vi "v5.5.vi"() -> ()   [LabVIEW 2018]
uses:
  <vilib>/DAQmx/read.llb/DAQmx Read (Analog 1D DBL NChan 1Samp).vi
  <extravilib>/ChannelInstances/Lossy Stream-c(a[.](c(dbl,dbl,dbl,dbl)),stamp,a[.](dbl),c(dbl,dbl,dbl,dbl,dbl,dbl,dbl))/Read With Abort.vi
  <extravilib>/ChannelInstances/High Speed Stream-c(a[.](c(dbl,dbl,dbl,dbl)),stamp,a[.](dbl),c(dbl,dbl,dbl,dbl,dbl,dbl,dbl))/_Read For Replicate.vi
  <extravilib>/ChannelInstances/Lossy Stream-c(a[.](c(dbl,dbl,dbl,dbl)),stamp,a[.](dbl),c(dbl,dbl,dbl,dbl,dbl,dbl,dbl))/Write With Abort.vi
  <extravilib>/ChannelInstances/Lossy Stream-c(a[.](c(dbl,dbl,dbl,dbl)),stamp,a[.](dbl),c(dbl,dbl,dbl,dbl,dbl,dbl,dbl))/EndpointRead.vi
  <extravilib>/ChannelInstances/Lossy Stream-c(a[.](c(dbl,dbl,dbl,dbl)),stamp,a[.](dbl),c(dbl,dbl,dbl,dbl,dbl,dbl,dbl))/Endpoint.vi
  <extravilib>/ChannelInstances/Lossy Stream-c(a[.](c(dbl,dbl,dbl,dbl)),stamp,a[.](dbl),c(dbl,dbl,dbl,dbl,dbl,dbl,dbl))/Instantiate.vi
  <extravilib>/ChannelInstances/Lossy Stream-c(a[.](c(dbl,dbl,dbl,dbl)),stamp,a[.](dbl),c(dbl,dbl,dbl,dbl,dbl,dbl,dbl))/)Channel.vi
  <resource>/ChannelSupport/_ChannelSupport/WaitIfNeeded.vi
  <extravilib>/ChannelInstances/High Speed Stream-c(a[.](c(dbl,dbl,dbl,dbl)),stamp,a[.](dbl),c(dbl,dbl,dbl,dbl,dbl,dbl,dbl))/Instantiate.vi
  <extravilib>/ChannelInstances/High Speed Stream-c(a[.](c(dbl,dbl,dbl,dbl)),stamp,a[.](dbl),c(dbl,dbl,dbl,dbl,dbl,dbl,dbl))/)Channel.vi
  <extravilib>/ChannelInstances/High Speed Stream-c(a[.](c(dbl,dbl,dbl,dbl)),stamp,a[.](dbl),c(dbl,dbl,dbl,dbl,dbl,dbl,dbl))/Abort Signal/Init Signal.vi
  <vilib>/Utility/file.llb/Write Delimited Spreadsheet (string).vi
  <vilib>/DAQmx/create/channels.llb/DAQmx Create Channel (AI-Temperature-Thermocouple).vi
  <vilib>/DAQmx/configure/timing.llb/DAQmx Timing (Sample Clock).vi
  <vilib>/DAQmx/miscellaneous.llb/DAQmx Fill In Error Info.vi
  <extravilib>/ChannelInstances/High Speed Stream-c(a[.](c(dbl,dbl,dbl,dbl)),stamp,a[.](dbl),c(dbl,dbl,dbl,dbl,dbl,dbl,dbl)).lvlib
  <resource>/objmgr/daqmx.rc
  <extravilib>/ChannelInstances/Lossy Stream-c(a[.](c(dbl,dbl,dbl,dbl)),stamp,a[.](dbl),c(dbl,dbl,dbl,dbl,dbl,dbl,dbl)).lvlib
panel:
  out "Equivalence Ratio":dbl
  out "Total Air Flow Required for Stoichiometric Combustion":dbl
  out "Mixture AFR":dbl
  out "Total Fuel Flow [g/s]":dbl
  out "Total Air Flow [g/s]":dbl
  in  "Rig Temperature Tab Box":enum32{"Rig Temps Live", "Alarm Thresholds"}(tab)
  out "Rig Temperatures":T1
  in  "Rig Alarm Thresholds":T1
  out "DAQ Current Time":timestamp format="%<%X>T"
  in  "UI Refresh Rate (Hz)":u32=1 min=1 max=500 step=1
  out "Line Pressures":T2(graph)
  in  "Boondoggle":dbl(slide) scale=0.0..10.0
  out "Line Temperatures":T2(graph)
  in  "Species List":string[][](table)=[["Custom", "9999999999"], ["Methanol", "6.47"], ["Butanol", "11.2"], ["Diesel", "14.5"], ["Gasoline", "14.7"], ["Propane", "15.67"], ["Methane", "13.19"], ["Hydrogen", "34.3"], ["Ammonia", "6.0466"], ["Pentane", "15.32"], ["Butane", "14.98"], ["Hexane", "15.24"], ["Ethanol", "9"], ["Empty (Not Used)", "0"]]
  in  "Lines Tab Control\n(Don't delete)":enum32{"Live Data", "AFR Info", "Setup Lines"}(tab)
  out "Flowrate Data":T3(array[cluster])
  out "AFR Display":T4(array[cluster])
  in  "Line Setup":T5(array[cluster])
  out "Actual Sample Rate":dbl
  out "Export Timestamp":timestamp format="%<%H:%M:%S>T"
  out "UI Timestamp":timestamp format="%<%X\n%x>T"
  in  "file path (dialog if empty)":path
  out "Export Loop Status":T6(ring)
  in  "Start Recording?":bool
  in  "Stop Recording?":bool
  out "Aquisition\nLoop Status":T7(ring)
  in  "OK Button":bool
  in  "DAQ Properties":cluster{"Sample Rate [Hz]":dbl}={"Sample Rate [Hz]"=1.0} {"Sample Rate [Hz]" min=1.0 max=500.0 step=1.0}
  # "Rig Temperatures [ °C]"
  # "Rig Alarm Thresholds [ °C]"
  # "Live \n Live Line Data"
  # "Air-to-Fuel Ratios for each Line"
  # "Line Setup"
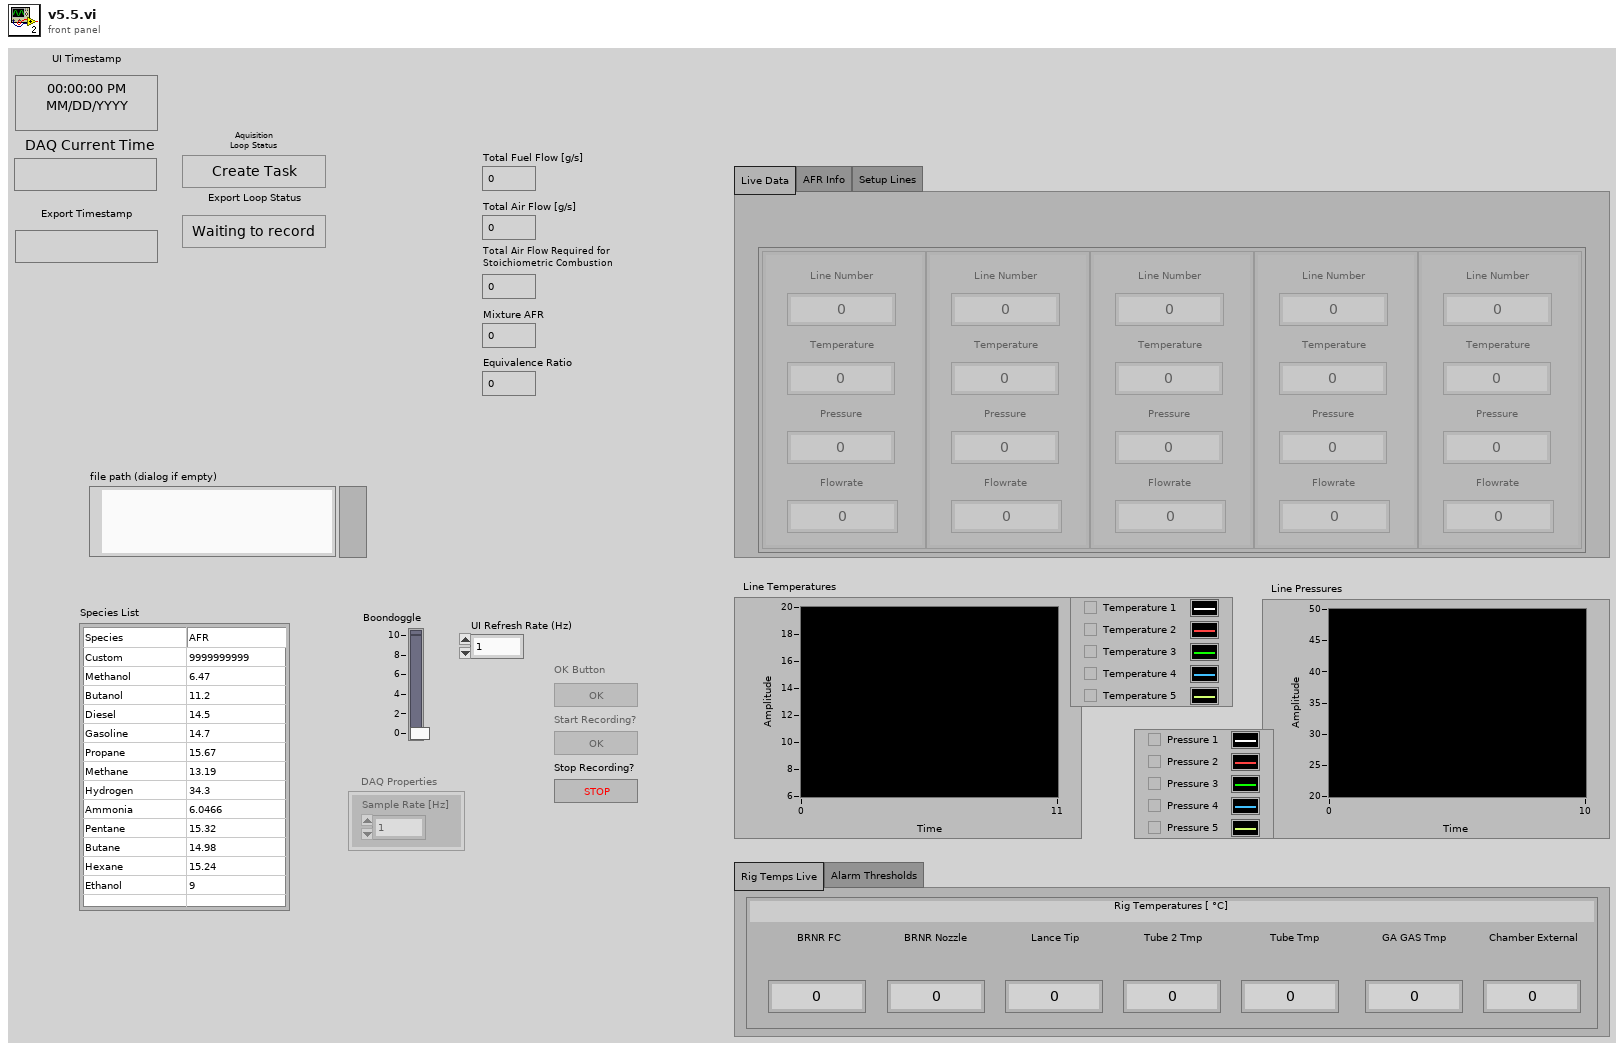
[diagram p1: front panel]
types:
  T1 = cluster{"BRNR FC":dbl, "BRNR Nozzle":dbl, "Lance Tip":dbl, "Tube 2 Tmp":dbl, "Tube Tmp":dbl, "GA GAS Tmp":dbl, "Chamber External":dbl}
  T2 = cluster{"[0]":dbl, "[1]":dbl, "[2]":dbl, "[3]":dbl, "[4]":dbl}
  T3 = cluster{"Line Number":dbl, "Temperature":dbl, "Pressure":dbl, "Flowrate":dbl}[]
  T4 = cluster{"Line Number":i32, "AFR":dbl, "Species":enum16{"Empty (Not used)", "Custom", "Air", "Methanol", "Ethanol", "Butanol", "Diesel", "Gasoline", "Propane", "Methane", "Hydrogen", "Pentane", "Butane", "Hexane"}}[]
  T5 = cluster{"Custom AFR":dbl, "Species":enum16{"Empty (Not used)", "Custom", "Air", "Methanol", "Ethanol", "Butanol", "Diesel", "Gasoline", "Propane", "Methane", "Hydrogen", "Pentane", "Butane", "Hexane"}}[]
  T6 = enum16{"Waiting to record", "Creating Spreadsheet", "Recording", "Finished Recording"}
  T7 = enum16{"Create Task", "Change Settings", "Check Settings", "Read Data", "End Task"}
  T8 = enum8{"Enabled", "Disabled", "Disabled and Grayed Out"}
  T9 = cluster{"Flowrate Data":cluster{"Line Number":dbl, "Temperature":dbl, "Pressure":dbl, "Flowrate":dbl}[], "Current Time":timestamp, "DAQmx Data":dbl[], "Rig Temperatures":cluster{"BRNR FC":dbl, "BRNR Nozzle":dbl, "Lance Tip":dbl, "Tube 2 Tmp":dbl, "Tube Tmp":dbl, "GA GAS Tmp":dbl, "Chamber External Temp":dbl}}
  T10 = cluster{"BRNR FC":dbl, "BRNR Nozzle":dbl, "Lance Tip":dbl, "Tube 2 Tmp":dbl, "Tube Tmp":dbl, "GA GAS Tmp":dbl, "Chamber External Temp":dbl}
  T11 = typedef "High Speed Stream-c(a[.](c(dbl,dbl,dbl,dbl)),stamp,a[.](dbl),c(dbl,dbl,dbl,dbl,dbl,dbl,dbl)).lvlib/)Channel.ctl" = refnum<queue>
  T12 = typedef "Lossy Stream-c(a[.](c(dbl,dbl,dbl,dbl)),stamp,a[.](dbl),c(dbl,dbl,dbl,dbl,dbl,dbl,dbl)).lvlib/)Channel.ctl" = refnum<queue>
  T13 = cluster{"Line":i32, "AFR":dbl, "Species":enum16{"Empty (Not used)", "Custom", "Air", "Methanol", "Ethanol", "Butanol", "Diesel", "Gasoline", "Propane", "Methane", "Hydrogen", "Pentane", "Butane", "Hexane"}}
  T14 = enum16{"Empty (Not used)", "Custom", "Air", "Methanol", "Ethanol", "Butanol", "Diesel", "Gasoline", "Propane", "Methane", "Hydrogen", "Pentane", "Butane", "Hexane"}
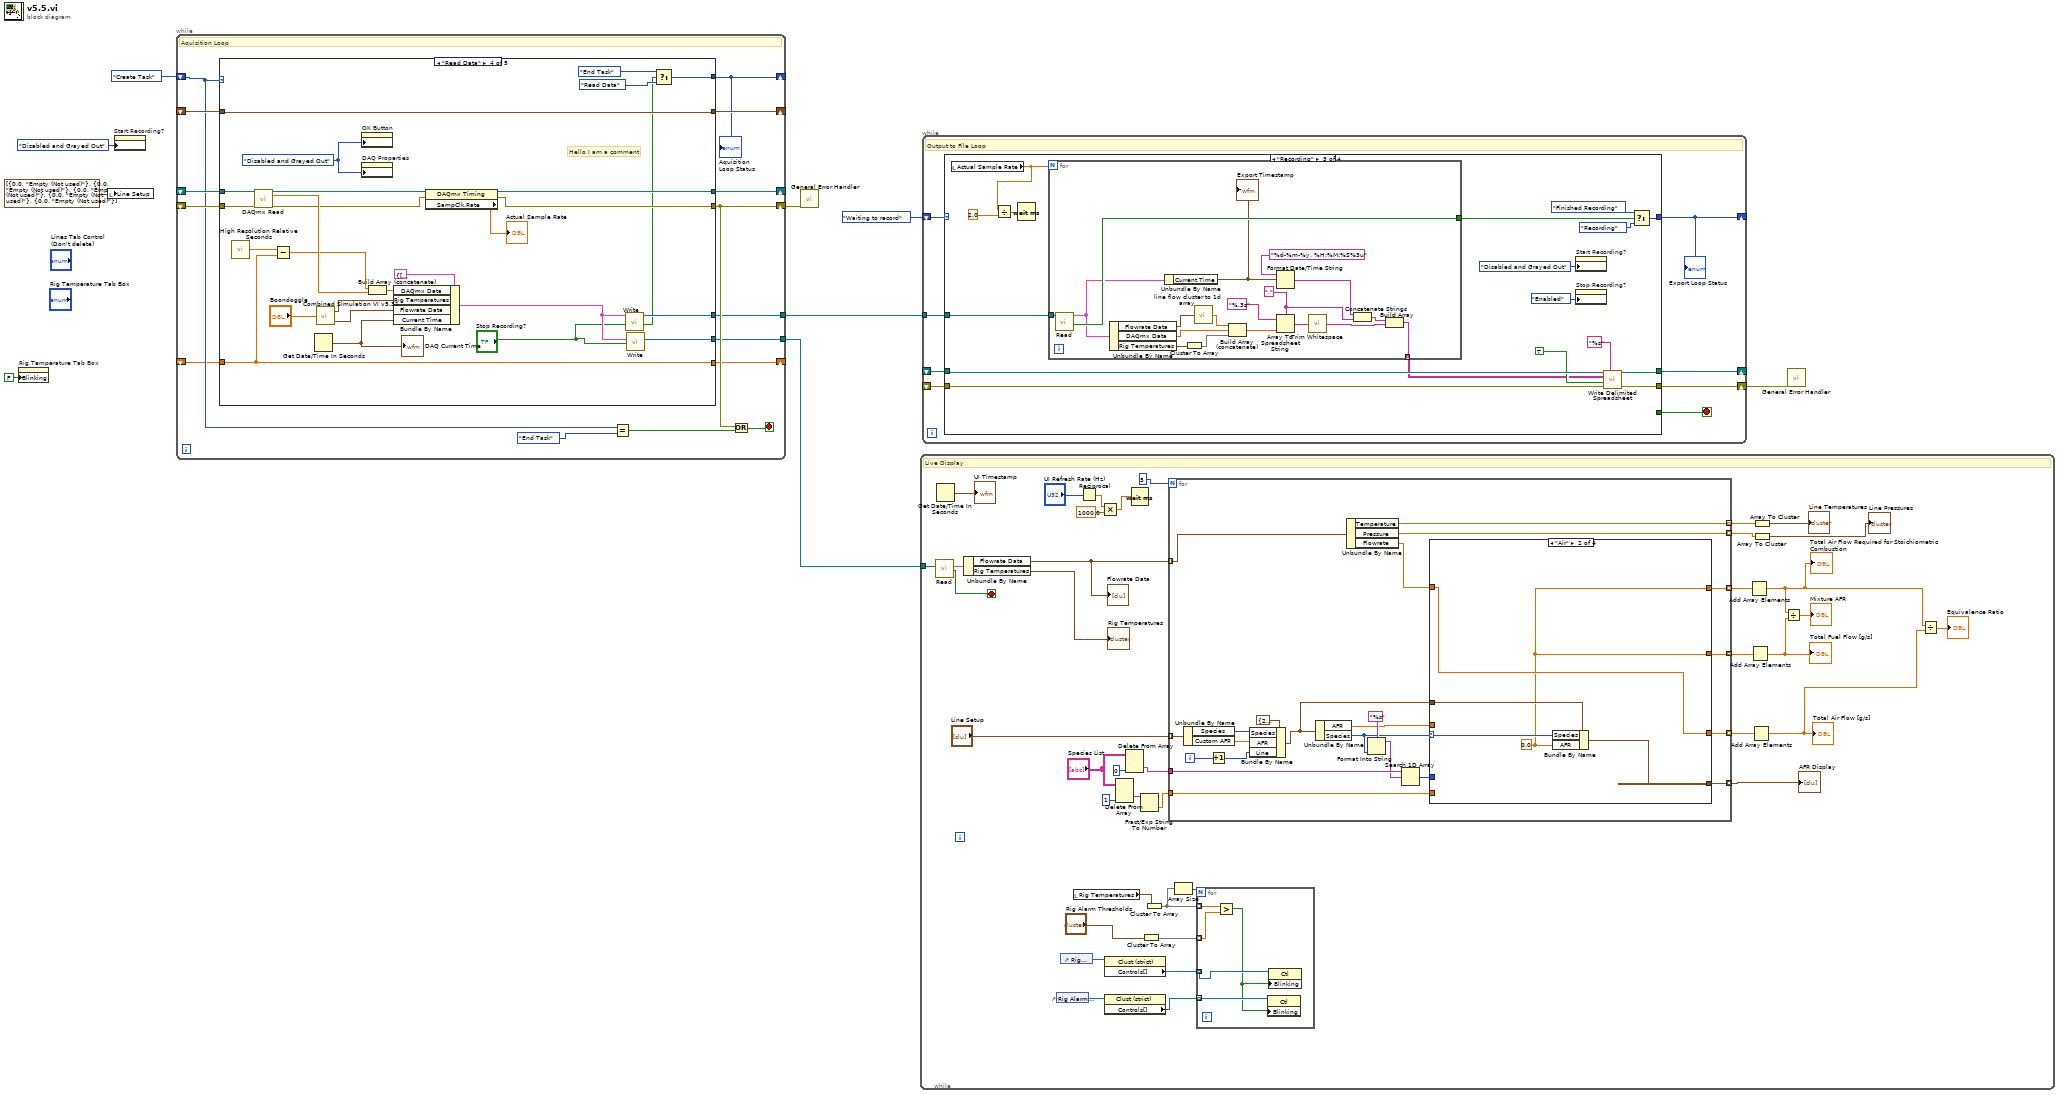
[diagram p0: block diagram]
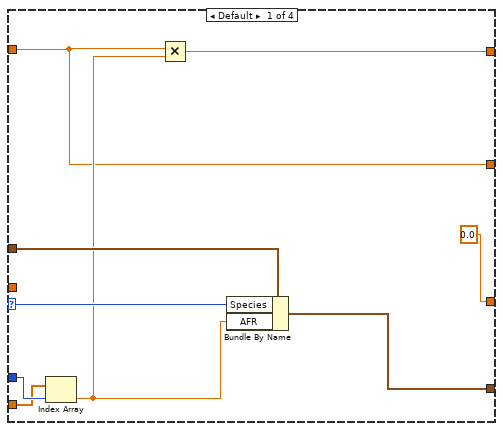
[diagram p2: hidden frame]
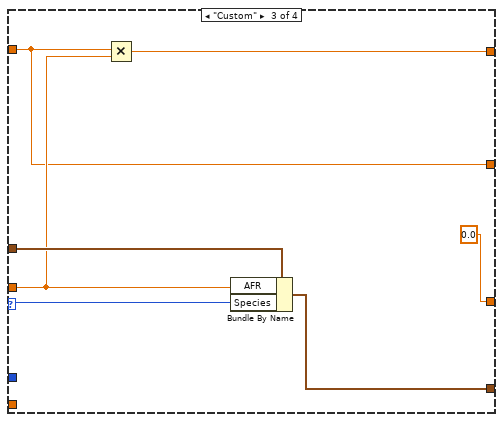
[diagram p3: hidden frame]
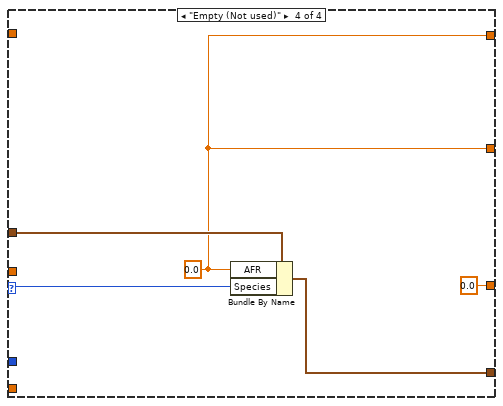
[diagram p4: hidden frame]
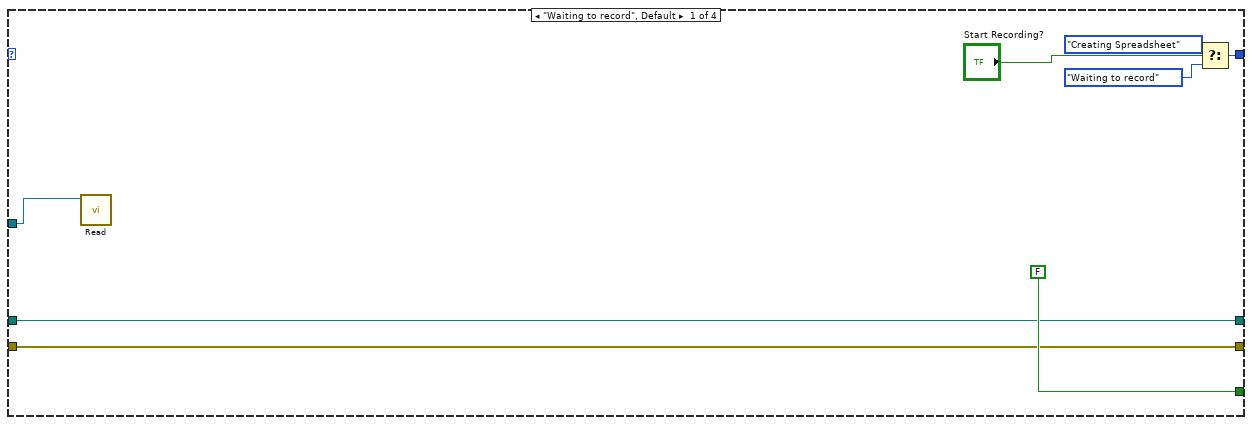
[diagram p5: hidden frame]
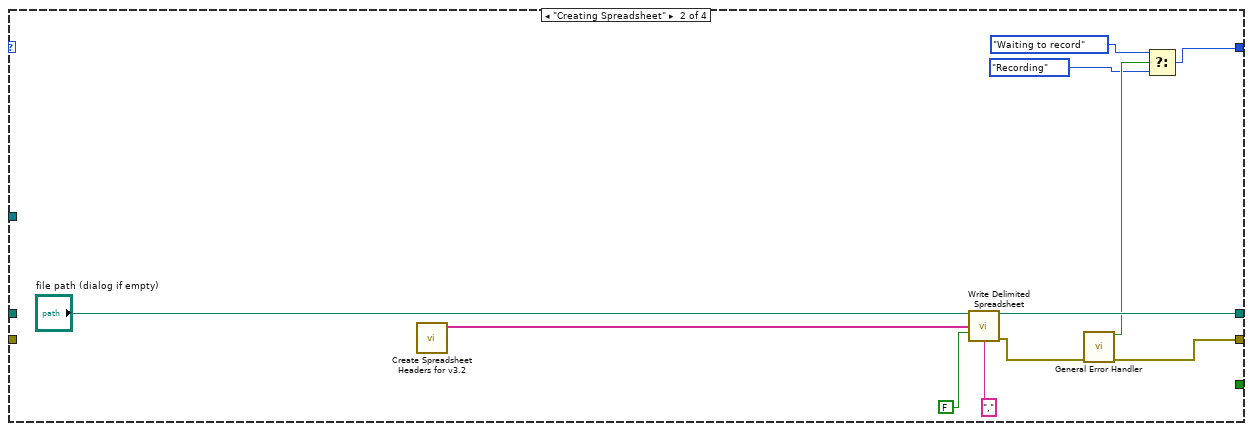
[diagram p6: hidden frame]
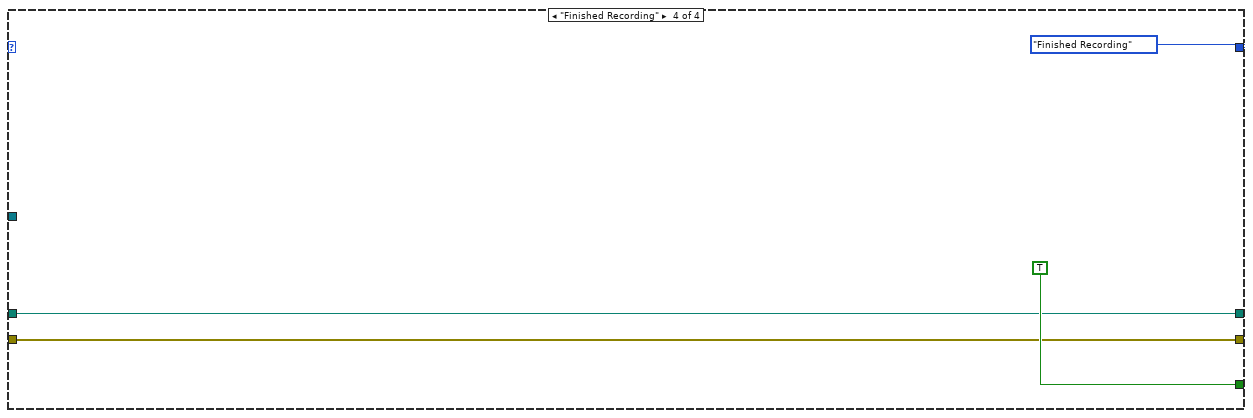
[diagram p7: hidden frame]
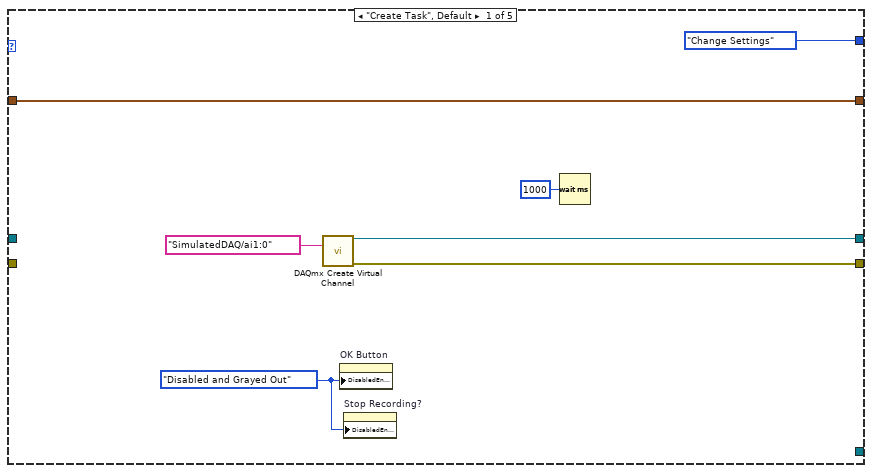
[diagram p8: hidden frame]
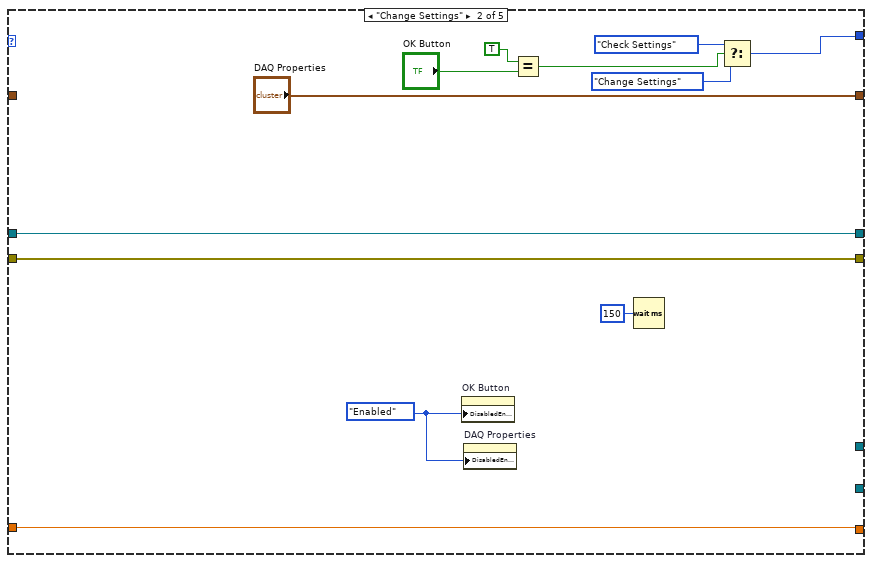
[diagram p9: hidden frame]
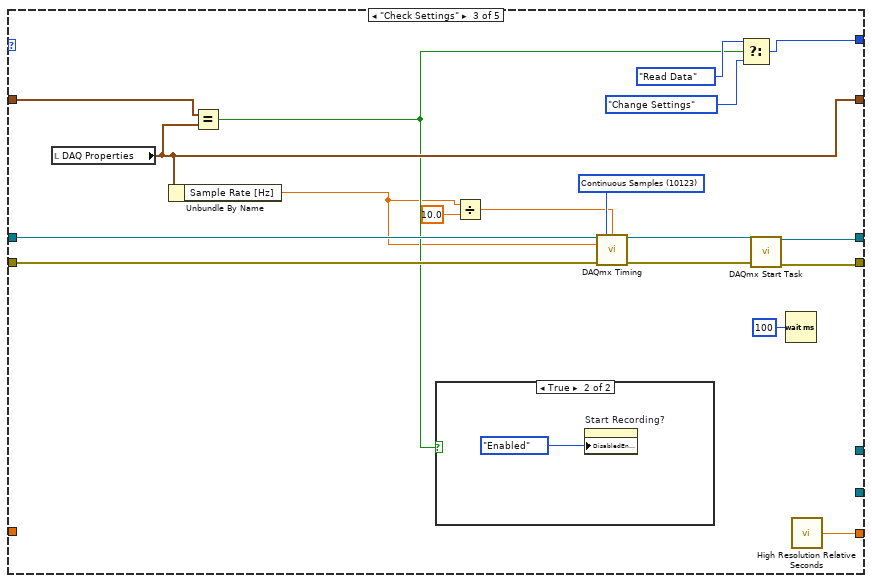
[diagram p10: hidden frame]
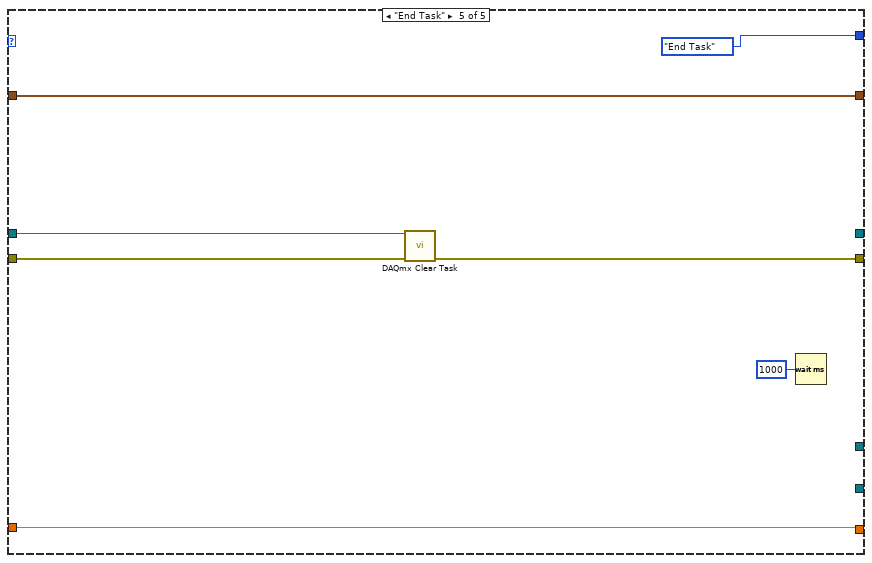
[diagram p12: hidden frame]
diagram:
  n1 = property on="Rig Temperature Tab Box" class="TabCtl (strict)"("Blinking"=FALSE) -> ()  [unwired: 2 in, 2 out]
  n2 = local write "Line Setup"(T5 [{"Custom AFR"=0.0, "Species"=enum."Empty (Not used)"}, {"Custom AFR"=0.0, "Species"=enum."Empty (Not used)"}, {"Custom AFR"=0.0, "Species"=enum."Empty (Not used)"}, {"Custom AFR"=0.0, "Species"=enum."Empty (Not used)"}, {"Custom AFR"=0.0, "Species"=enum."Empty (Not used)"}] ("Line Setup 2")) -> ()
  n3 = property on="Start Recording?" class="Bool"("DisabledEnum"=T8."Disabled and Grayed Out" ("Disabled")) -> ()  [unwired: 2 in, 2 out]
  n4 = while {
    shift-right: [w19] -> _
    shift-left: T7."Create Task" -> [w15]
    shift-right: [w24] -> _
    shift-left: _ -> [w22]
    shift-right: [w18] -> w5
    shift-left: _ -> [w21]
    shift-right: [w23] -> _
    shift-left: _ -> [w20]
    tunnel: [w14] -> w7
    tunnel: [w12] -> w3
    shift-right: [w10] -> _
    shift-left: _ -> [w11]
    stop <- w13 stop-if-true
    # "Aquisition Loop"
    n5 = case shown="\"Read Data\"" w15 {
      tunnel: [w31 w43 w51 w76 _] -> w24
      tunnel: [w30 w42 w50 w77 w96] -> w18
      tunnel: [T7."Change Settings" w36 w57 w85 T7."End Task"] -> w19
      tunnel: [w27 "DAQ Properties" w54 w87 w95] -> w23
      tunnel: w22 -> [_ w43 w56 w89 w93]
      tunnel: w21 -> [_ w42 w55 w88 w92]
      tunnel: w20 -> [w27 _ w61 w87 w95]
      tunnel: [_ _ _ w81 _] -> w14
      tunnel: [_ w32 w44 w72 w90] -> w10
      tunnel: w11 -> [_ w32 _ w72 w90]
      tunnel: [_ _ _ w69 _] -> w12
      frame "Create Task", Default {
        w25 = T8."Disabled and Grayed Out" ("Disabled")
        n6 = call-poly <vilib>:"DAQmx Create Virtual Channel.vi"("physical channels"=tag "SimulatedDAQ/ai1:0") -> ("task out"=w31:refnum<k21>, "error out"=w30:errorcluster)  [unwired: 13 in]
        n7 = property on="OK Button" class="Bool"("DisabledEnum"=w25) -> ()  [unwired: 2 in, 2 out]
        n8 = property on="Stop Recording?" class="Bool"("DisabledEnum"=w25) -> ()  [unwired: 2 in, 2 out]
        n9 = Wait (ms)(milliseconds to wait=u32 1000) -> ()  [unwired: 1 out]
      }
      frame "Change Settings" {
        w33 = T8."Enabled" ("Disabled")
        n10 = property on="OK Button" class="Bool"("DisabledEnum"=w33) -> ()  [unwired: 2 in, 2 out]
        n11 = property on="DAQ Properties" class="Clust (strict)"("DisabledEnum"=w33) -> ()  [unwired: 2 in, 2 out]
        n12 = Equal?(x=TRUE, y="OK Button") -> (x = y?=w38:bool)
        n13 = Wait (ms)(milliseconds to wait=u32 150) -> ()  [unwired: 1 out]
        n14 = Select(t=T7."Check Settings", s=w38, f=T7."Change Settings") -> (s? t:f=w36:T7)
      }
      frame "Check Settings" {
        w49 = 10123 items=["Finite Samples"=10178, "Continuous Samples"=10123, "Hardware Timed Single Point"=12522] ("sample mode")
        n15 = local read "DAQ Properties"() -> (w54:cluster{"Sample Rate [Hz]":dbl})
        n16 = Unbundle By Name(w54) -> ("Sample Rate [Hz]"=w46:dbl)
        n17 = Equal?(x=w61, y=w54) -> (x = y?=w48:bool)
        n18 = case shown="True" w48 {
          frame False {
          }
          frame True {
            n19 = property on="Start Recording?" class="Bool"("DisabledEnum"=T8."Enabled" ("Disabled")) -> ()  [unwired: 2 in, 2 out]
          }
        }
        n20 = Divide(x=w46, y=10.0) -> (x/y=w45:dbl)
        n21 = call-poly <vilib>:"DAQmx Timing.vi"("task/channels in"=w56, "sample mode"=w49, "samples per channel"=w45, "rate"=w46, "error in"=w55) -> ("task out"=w53:refnum<k21>, "error out"=w52:errorcluster)  [unwired: 9 in]
        n22 = Select(t=T7."Read Data", s=w48, f=T7."Change Settings") -> (s? t:f=w57:T7)
        n23 = call <vilib>:"DAQmx Start Task.vi"("task/channels in"=w53, "error in"=w52) -> ("task out"=w51:refnum<k21>, "error out"=w50:errorcluster)  [unwired: 12 in]
        n24 = Wait (ms)(milliseconds to wait=u32 100) -> ()  [unwired: 1 out]
        n25 = call <vilib>:"High Resolution Relative Seconds.vi"() -> ("relative seconds"=w44:dbl)
      }
      frame "Read Data" {
        w80 = T8."Disabled and Grayed Out" ("Disabled")
        # "Hello I am a comment"
        n26 = call <vilib>:"High Resolution Relative Seconds.vi"() -> ("relative seconds"=w74:dbl)
        n27 = call-poly <vilib>:"DAQmx Read.vi"("task/channels in"=w89, "error in"=w88) -> ("task out"=w78:refnum<k21>, "data"=w83:dbl[], "error out"=w75:errorcluster)  [unwired: 11 in]
        n28 = Subtract(x=w74, y=w72) -> (x-y=w73:dbl)
        n29 = Get Date/Time In Seconds() -> (seconds since 1Jan1904=w64:timestamp)
        "DAQ Current Time" <- w64
        n30 = call "Combined Simulation VI v5.31.vi"("Boondoggle Input"="Boondoggle") -> ("Rig Temperatures Cluster"=w63:T10, "Line Data (Array of Clusters)"=w65:T3)
        n31 = property on="OK Button" class="Bool"("DisabledEnum"=w80) -> ()  [unwired: 2 in, 2 out]
        n32 = property on="DAQ Properties" class="Clust (strict)"("DisabledEnum"=w80) -> ()  [unwired: 2 in, 2 out]
        n33 = Build Array (concatenate)(w73, w83) -> (w67:dbl[])
        n34 = Bundle By Name(cluster=T9 {"Flowrate Data"=[{"Line Number"=1.0, "Temperature"=17.480721541683437, "Pressure"=24.0, "Flowrate"=0.0}, {"Line Number"=2.0, "Temperature"=21.850901927104296, "Pressure"=30.0, "Flowrate"=0.0}, {"Line Number"=3.0, "Temperature"=26.221082312525155, "Pressure"=36.0, "Flowrate"=0.0}, {"Line Number"=4.0, "Temperature"=30.591262697946018, "Pressure"=42.00000000000001, "Flowrate"=0.0}, {"Line Number"=5.0, "Temperature"=34.96144308336687, "Pressure"=48.0, "Flowrate"=0.0}], "Current Time"=timestamp(0 s since 1904-01-01), "DAQmx Data"=[], "Rig Temperatures"={"BRNR FC"=0.0, "BRNR Nozzle"=0.0, "Lance Tip"=0.0, "Tube 2 Tmp"=0.0, "Tube Tmp"=0.0, "GA GAS Tmp"=0.0, "Chamber External Temp"=0.0}}, "DAQmx Data"=w67, "Rig Temperatures"=w63, "Flowrate Data"=w65, "Current Time"=w64) -> (w79:T9)
        n35 = property class="DAQmx Timing"(reference=w78, error in=w75) -> (reference out=w76:refnum<k21>, error out=w77:errorcluster, "SampClk.Rate"=→"Actual Sample Rate":dbl)
        n36 = call <extravilib>:"Write.vi"("last element? (F)"="Stop Recording?", "element"=w79) -> ("done?"=w68:bool, "channel"=w81:T11)  [unwired: 7 in, 1 out]
        n37 = call <extravilib>:"Write.vi"("last element? (F)"="Stop Recording?", "element"=w79) -> ("channel"=w69:T12)  [unwired: 7 in, 2 out]
        n38 = Select(t=T7."End Task", s=w68, f=T7."Read Data") -> (s? t:f=w85:T7)
      }
      frame "End Task" {
        n39 = call <vilib>:"DAQmx Clear Task.vi"("task in"=w93, "error in"=w92) -> ("error out"=w96:errorcluster)  [unwired: 13 in]
        n40 = Wait (ms)(milliseconds to wait=u32 1000) -> ()  [unwired: 1 out]
      }
    }
    "Aquisition\nLoop Status" <- w19
    n41 = Equal?(x=w15, y=T7."End Task") -> (x = y?=w16:bool)
    n42 = Or(x=w18, y=w16) -> (x .or. y?=w13:bool)
  }
  n43 = call <vilib>:"General Error Handler.vi"("error in (no error)"=w5) -> ()  [unwired: 10 in, 5 out]
  n44 = while {
    tunnel: w3 -> [w135]
    stop <- w132 stop-if-true
    # "Live Display"
    n45 = call <extravilib>:"Read.vi"("channel"=w135) -> ("last element?"=w132:bool, "element"=w134:T9)  [unwired: 5 in, 4 out]
    n46 = Get Date/Time In Seconds() -> (seconds since 1Jan1904=→"UI Timestamp":timestamp)
    n47 = Unbundle By Name(w134) -> ("Flowrate Data"=w109:T3, "Rig Temperatures"=→"Rig Temperatures":T10)
    "Flowrate Data" <- w109
    n48 = control-ref of="Rig Alarm Thresholds"() -> (w98:refnum<vi>)
    n49 = control-ref of="Rig Temperatures"() -> (w100:refnum<vi>)
    n50 = local read "Rig Temperatures"() -> (w104:T1)
    n51 = Reciprocal(x="UI Refresh Rate (Hz)") -> (1/x=w129:dbl)
    n52 = Multiply(x=w129, y=1000.0) -> (x*y=w128:dbl)
    n53 = property class="Clust (strict)"(reference=w98) -> ("Controls[]"=w97:refnum<vi>[])  [unwired: 1 in, 2 out]
    n54 = property class="Clust (strict)"(reference=w100) -> ("Controls[]"=w99:refnum<vi>[])  [unwired: 1 in, 2 out]
    n55 = Delete From Array(array="Species List", index (col)=1 ("disabled index (col)")) -> (deleted portion=w124:string[])  [unwired: 2 in, 1 out]
    n56 = Delete From Array(array="Species List", index (col)=0) -> (deleted portion=w123:string[])  [unwired: 2 in, 1 out]
    n57 = Wait (ms)(milliseconds to wait=w128) -> ()  [unwired: 1 out]
    n58 = Fract/Exp String To Number(string=w124) -> (number=w125:dbl[])  [unwired: 3 in, 1 out]
    n59 = Cluster To Array(cluster="Rig Alarm Thresholds") -> (array=w103:dbl[])
    n60 = Cluster To Array(cluster=w104) -> (array=w101:dbl[])
    n61 = for {
      N: 5 -> [_]
      tunnel: w123 -> [w162]
      tunnel: w125 -> [w159]
      tunnel: "Line Setup" -> [w152] mode=indexing
      tunnel: [w149] -> w127 mode=indexing
      tunnel: w109 -> [w143] mode=indexing
      tunnel: [w148] -> w117 mode=indexing
      tunnel: [w147] -> w114 mode=indexing
      tunnel: [w145] -> w112 mode=indexing
      tunnel: [w144] -> w111 mode=indexing
      tunnel: [w142] -> w110 mode=indexing
      i -> [w151]
      n62 = Unbundle By Name(w152) -> ("Species"=w156:T14, "Custom AFR"=w155:dbl)
      n63 = Increment(x=w151) -> (x+1=w153:i32)
      n64 = Bundle By Name(cluster=T13 {"Line"=2, "AFR"=1.0, "Species"=enum."Hydrogen"} ("AFR Inputs"), "Species"=w156, "AFR"=w155, "Line"=w153) -> (w150:T13)
      n65 = Unbundle By Name(w150) -> ("AFR"=w160:dbl, "Species"=w157:T14)
      n66 = Unbundle By Name(w143) -> ("Temperature"=w148:dbl, "Pressure"=w147:dbl, "Flowrate"=w146:dbl)
      n67 = Format Into String(format string="%s", w157) -> (resulting string=w161:string)  [unwired: 2 in, 1 out]
      n68 = Search 1D Array(1D array=w162, element=w161) -> (index of element=w158:i32)  [unwired: 1 in]
      n69 = case shown="\"Air\"" w157 {
        selector: w157 -> [w170 w177 w182 w187]
        tunnel: w160 -> [_ _ w180 _]
        tunnel: w159 -> [w171 _ _ _]
        tunnel: w158 -> [w172 _ _ _]
        tunnel: [w168 w176 w184 w189] -> w149
        tunnel: w150 -> [w169 w175 w183 w188]
        tunnel: w146 -> [w164 w174 w178 _]
        tunnel: [w166 w173 w179 w186] -> w145
        tunnel: [w164 w173 w178 w186] -> w144
        tunnel: [0.0 ("Flowrate") w174 0.0 ("Flowrate") 0.0 ("Flowrate")] -> w142
        frame Default {
          n70 = Index Array(array=w171, index=w172) -> (element=w167:dbl)
          n71 = Multiply(x=w164, y=w167) -> (x*y=w166:dbl)
          n72 = Bundle By Name(cluster=w169, "Species"=w170, "AFR"=w167) -> (w168:T13)
        }
        frame "Air" {
          w173 = 0.0 ("AFR")
          n73 = Bundle By Name(cluster=w175, "Species"=w177, "AFR"=w173) -> (w176:T13)
        }
        frame "Custom" {
          n74 = Multiply(x=w178, y=w180) -> (x*y=w179:dbl)
          n75 = Bundle By Name(cluster=w183, "AFR"=w180, "Species"=w182) -> (w184:T13)
        }
        frame "Empty (Not used)" {
          w186 = 0.0 ("AFR")
          n76 = Bundle By Name(cluster=w188, "AFR"=w186, "Species"=w187) -> (w189:T13)
        }
      }
    }
    "AFR Display" <- w127
    n77 = Array Size(array=w101) -> (size(s)=w102:i32)
    n78 = for {
      N: w102 -> [_]
      tunnel: w103 -> [w140] mode=indexing
      tunnel: w101 -> [w141] mode=indexing
      tunnel: w99 -> [w138] mode=indexing
      tunnel: w97 -> [w139] mode=indexing
      n79 = Greater?(x=w141, y=w140) -> (0:w137:bool)
      n80 = property on="Property Node" class="Ctl"(reference=w139, "Blinking"=w137) -> ()  [unwired: 1 in, 2 out]
      n81 = property on="Property Node" class="Ctl"(reference=w138, "Blinking"=w137) -> ()  [unwired: 1 in, 2 out]
    }
    n82 = Add Array Elements(numeric array=w112) -> (sum=w107:dbl)
    "Total Air Flow Required for Stoichiometric Combustion" <- w107
    n83 = Add Array Elements(numeric array=w111) -> (sum=w115:dbl)
    "Total Fuel Flow [g/s]" <- w115
    n84 = Add Array Elements(numeric array=w110) -> (sum=w106:dbl)
    "Total Air Flow [g/s]" <- w106
    n85 = Array To Cluster(array=w114) -> (cluster=→"Line Pressures":T2)
    n86 = Array To Cluster(array=w117) -> (cluster=→"Line Temperatures":T2)
    n87 = Divide(x=w107, y=w115) -> (x/y=→"Mixture AFR":dbl)
    n88 = Divide(x=w107, y=w106) -> (x/y=→"Equivalence Ratio":dbl)
  }
  n89 = while {
    shift-right: [w197] -> _
    shift-left: T6."Waiting to record" -> [w196]
    tunnel: w7 -> [w194]
    shift-right: [w192] -> _
    shift-left: _ -> [w193]
    shift-right: [w191] -> w6
    shift-left: _ -> [w190]
    stop <- w195 stop-if-true
    # "Output to File Loop"
    n90 = case shown="\"Recording\"" w196 {
      tunnel: [w202 w208 w232 T6."Finished Recording"] -> w197
      tunnel: [FALSE _ _ TRUE] -> w195
      tunnel: w194 -> [w198 _ w229 _]
      tunnel: w193 -> [w200 _ w226 w253]
      tunnel: [w200 w216 w227 w253] -> w192
      tunnel: [w199 w210 w222 w252] -> w191
      tunnel: w190 -> [w199 _ w225 w252]
      frame "Waiting to record", Default {
        n91 = call <extravilib>:"Read.vi"("channel"=w198) -> ()  [unwired: 6 in, 5 out]
        n92 = Select(t=T6."Creating Spreadsheet", s="Start Recording?", f=T6."Waiting to record") -> (s? t:f=w202:T6)
      }
      frame "Creating Spreadsheet" {
        n93 = call "Create Spreadsheet Headers for v3.2.vi"() -> ("Array"=w215:string[])  [unwired: 11 in]
        n94 = call-poly <vilib>:"Write Delimited Spreadsheet.vi"("file path (dialog if empty)"="file path (dialog if empty)", "1D data"=w215, "append to file? (new file:F)"=FALSE, "delimiter (\\t)"="," ("delimiter (\\t)")) -> ("new file path (Not A Path if cancelled)"=w216:path, "error out"=w211:errorcluster)  [unwired: 10 in]
        n95 = call <vilib>:"General Error Handler.vi"("error in (no error)"=w211) -> ("error?"=w209:bool, "error out"=w210:errorcluster)  [unwired: 10 in, 3 out]
        n96 = Select(t=T6."Waiting to record", s=w209, f=T6."Recording") -> (s? t:f=w208:T6)
      }
      frame "Recording" {
        n97 = local read "Actual Sample Rate"() -> (w218:dbl)
        n98 = Divide(x=w218, y=2.0) -> (x/y=w217:dbl)
        n99 = Wait (ms)(milliseconds to wait=w217) -> ()  [unwired: 1 out]
        n100 = for {
          N: w218 -> [_]
          tunnel: w229 -> [w250]
          tunnel: [w249] -> w228
          tunnel: [w234] -> w220 mode=indexing
          w239 = "," ("delimiter (Tab)")
          n101 = call <extravilib>:"Read.vi"("channel"=w250) -> ("done?"=w249:bool, "element"=w247:T9)  [unwired: 6 in, 3 out]
          n102 = Unbundle By Name(w247) -> ("Flowrate Data"=w248:T3, "DAQmx Data"=w245:dbl[], "Rig Temperatures"=w251:T10)
          n103 = Unbundle By Name(w247) -> ("Current Time"=w240:timestamp)
          "Export Timestamp" <- w240
          n104 = Cluster To Array(cluster=w251) -> (array=w246:dbl[])
          n105 = call "line flow cluster to 1d array.vi"("Flowrate Data"=w248) -> ("Array"=w244:dbl[])
          n106 = Build Array (concatenate)(w244, w245, w246) -> (w237:dbl[])
          n107 = Format Date/Time String(time format string (%c)="%d-%m-%y, %H:%M:%S%3u", seconds (now)=w240) -> (date/time string=w238:string)  [unwired: 1 in]
          n108 = Array To Spreadsheet String(delimiter (Tab)=w239, array=w237, 3:"%.3s" ("format string")) -> (spreadsheet string=w243:string)
          n109 = call <vilib>:"Trim Whitespace.vi"("string"=w243) -> ("trimmed string"=w235:string)  [unwired: 1 in]
          n110 = Concatenate Strings(w238, w239) -> (w236:string)
          n111 = Build Array(w236, w235) -> (w234:string[])
        }
        n112 = property on="Start Recording?" class="Bool"("DisabledEnum"=T8."Disabled and Grayed Out" ("Disabled")) -> ()  [unwired: 2 in, 2 out]
        n113 = property on="Stop Recording?" class="Bool"("DisabledEnum"=T8."Enabled" ("Disabled")) -> ()  [unwired: 2 in, 2 out]
        n114 = call-poly <vilib>:"Write Delimited Spreadsheet.vi"("file path (dialog if empty)"=w226, "format (%s)"="%s", "2D data"=w220, "append to file? (new file:F)"=TRUE, "error in (no error)"=w225) -> ("new file path (Not A Path if cancelled)"=w227:path, "error out"=w222:errorcluster)  [unwired: 9 in]
        n115 = Select(t=T6."Finished Recording", s=w228, f=T6."Recording") -> (s? t:f=w232:T6)
      }
      frame "Finished Recording" {
      }
    }
    "Export Loop Status" <- w197
  }
  n116 = call <vilib>:"General Error Handler.vi"("error in (no error)"=w6) -> ()  [unwired: 10 in, 5 out]
